vi "CCImageToDcmPopulateDataset.vi"(8 "error in (no error)":errorcluster, 11 "Dataset":refnum<k24>) -> (0 "error out":errorcluster, 3 ".NET Refnum out":refnum<k24>)   [LabVIEW 2013, in "main.lvlib" / "ClearCanvasLibrary.lvlib"]
uses:
  ClearCanvasLibrary.lvlib
  C:/Users/Simon/SkyDrive/LabView/2013/DM2020/DICOM/ClearCanvasNewBuild/ClearCanvas.Dicom.dll
  ClearCanvasNewBuild/ClearCanvas.Dicom.dll
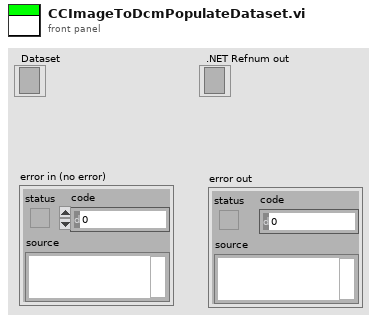
[diagram p1: front panel]
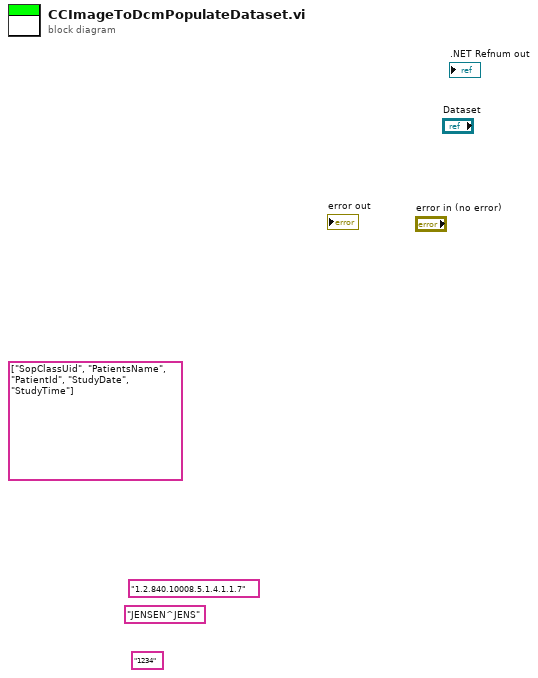
[diagram p0: block diagram]
diagram:
  (unwired) "1.2.840.10008.5.1.4.1.1.7" ("element")
  (unwired) string[] ["SopClassUid", "PatientsName", "PatientId", "StudyDate", "StudyTime"]
  (unwired) "1234" ("name")
  (unwired) "JENSEN^JENS" ("name")
